vi "Demo of affinity propagation clustering algorithm.vi"() -> ()   [LabVIEW 2020]
doc: "An algorithm that exchanges messages about the similarity of pairs of data points speeds identification of representative examples in a complex data set, such as genes in DNA data."
uses:
  PLAIYDISPLAY/Display/Classification/2D/Predicted/Controls/PredictedParameter.ctl
  PLAIYDISPLAY/Display/_Controls/Style.ctl
  Model/Unsupervised/Cluster/AffinityPropagation/Controls/affinity_propagation_params.ctl
  Model/Unsupervised/Cluster/AffinityPropagation/AffinityPropagation.lvclass
  C:/Users/cipop/TDF Dropbox/2_Technologies de France/1 - Services et Etudes/PLAIY/2 - DEV/PLAIYLAB/code/Model/Model.lvclass
  Model/Unsupervised/Cluster/AffinityPropagation/AffinityPropagation.vi
  Preproc/Objet/3 - Model selection and evaluation/3.3 - Metrics and scoring/silhouette_score/Silhouette_Score.vi
  Preproc/Objet/3 - Model selection and evaluation/3.3 - Metrics and scoring/homogeneity_score/Homogeneity_Score.vi
  Preproc/Objet/3 - Model selection and evaluation/3.3 - Metrics and scoring/completeness_score/Completeness_Score.vi
  Preproc/Objet/3 - Model selection and evaluation/3.3 - Metrics and scoring/v_measure_score/V_Measure_Score.vi
  Preproc/Objet/3 - Model selection and evaluation/3.3 - Metrics and scoring/adjusted_rand_score/Adjusted_Rand_Score.vi
  Preproc/Objet/3 - Model selection and evaluation/3.3 - Metrics and scoring/adjusted_mutual_info_score/Adjusted_Mutual_Info_Score.vi
panel:
  in  "Local":T1
  out "Silhouette Coefficient":string
  out "Adjusted Mutual Information":string
  out "Adjusted Rand Index":string
  out "V-measure":string
  out "Completeness":string
  out "Homogeneity":string
  out "error out":errorcluster
  out "Plot":cluster{"X":dbl[], "Y":dbl[]}[](graph) caption="Estimated number of cluster: 3"
  out "labels":dbl[](array[numeric])
  out "n_clusters_":i32
  out "cluster_centers_indices":dbl[](array[numeric])
  in  "error in (no error) 2":errorcluster caption="entrée d'erreur (pas d'erreur)"
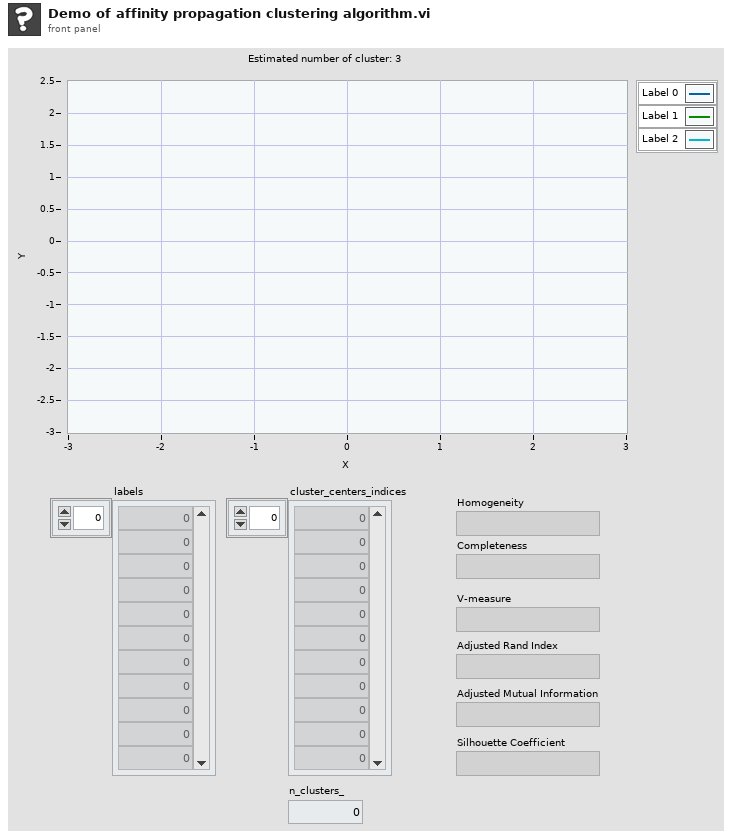
[diagram p1: front panel]
types:
  T1 = cluster{"X":dbl[][], "labels_true":dbl[], "labels_":dbl[]}
  T2 = cluster{"n_samples":i32[], "n_features":u32, "centers":i32[][], "cluster_std":dbl[], "centermin":dbl, "centermax":dbl, "shuffle":bool, "random_state":i32, "Returns":string}
  T3 = typedef "affinity_propagation_params.ctl" = cluster{"damping":dbl, "max_iter":i32, "convergence_iter":i32, "copy":bool, "preference":cluster{"preference_type":string, "preference_list":dbl[], "preference_float":dbl}, "affinity":string, "verbose":bool, "random_state":i32}
  T4 = typedef "Style.ctl" = enum16{"Empty circle", "Full circle", "Empty square", "Full square", "Cross"}
  T5 = typedef "PredictedParameter.ctl" = cluster{"Plot":refnum<vi>, "Data":cluster{"X":dbl[][], "Predict":dbl[][]}, "Indexe":cluster{"X":i32, "Y":i32}, "Point Property":cluster{"Style":T4, "Label Color":u32[]}}
  T6 = cluster{"metric":string, "sample_size":string, "random_state":i32}
  T7 = cluster{" 4DArray":cluster{"1":string[][], "2":string[][]}[], " 3DArray":cluster{"Tableau":string[][]}[], "Sparse Matrix 2DArray":string[][], " 2DArray":string[][], " 1DArray":string[]}
  T8 = typedef "affinity_propagation_attributes.ctl" = cluster{"cluster_centers_indices_":dbl[], "cluster_centers_":dbl[][], "labels_":dbl[], "affinity_matrix_":dbl[][], "n_iter_":dbl}
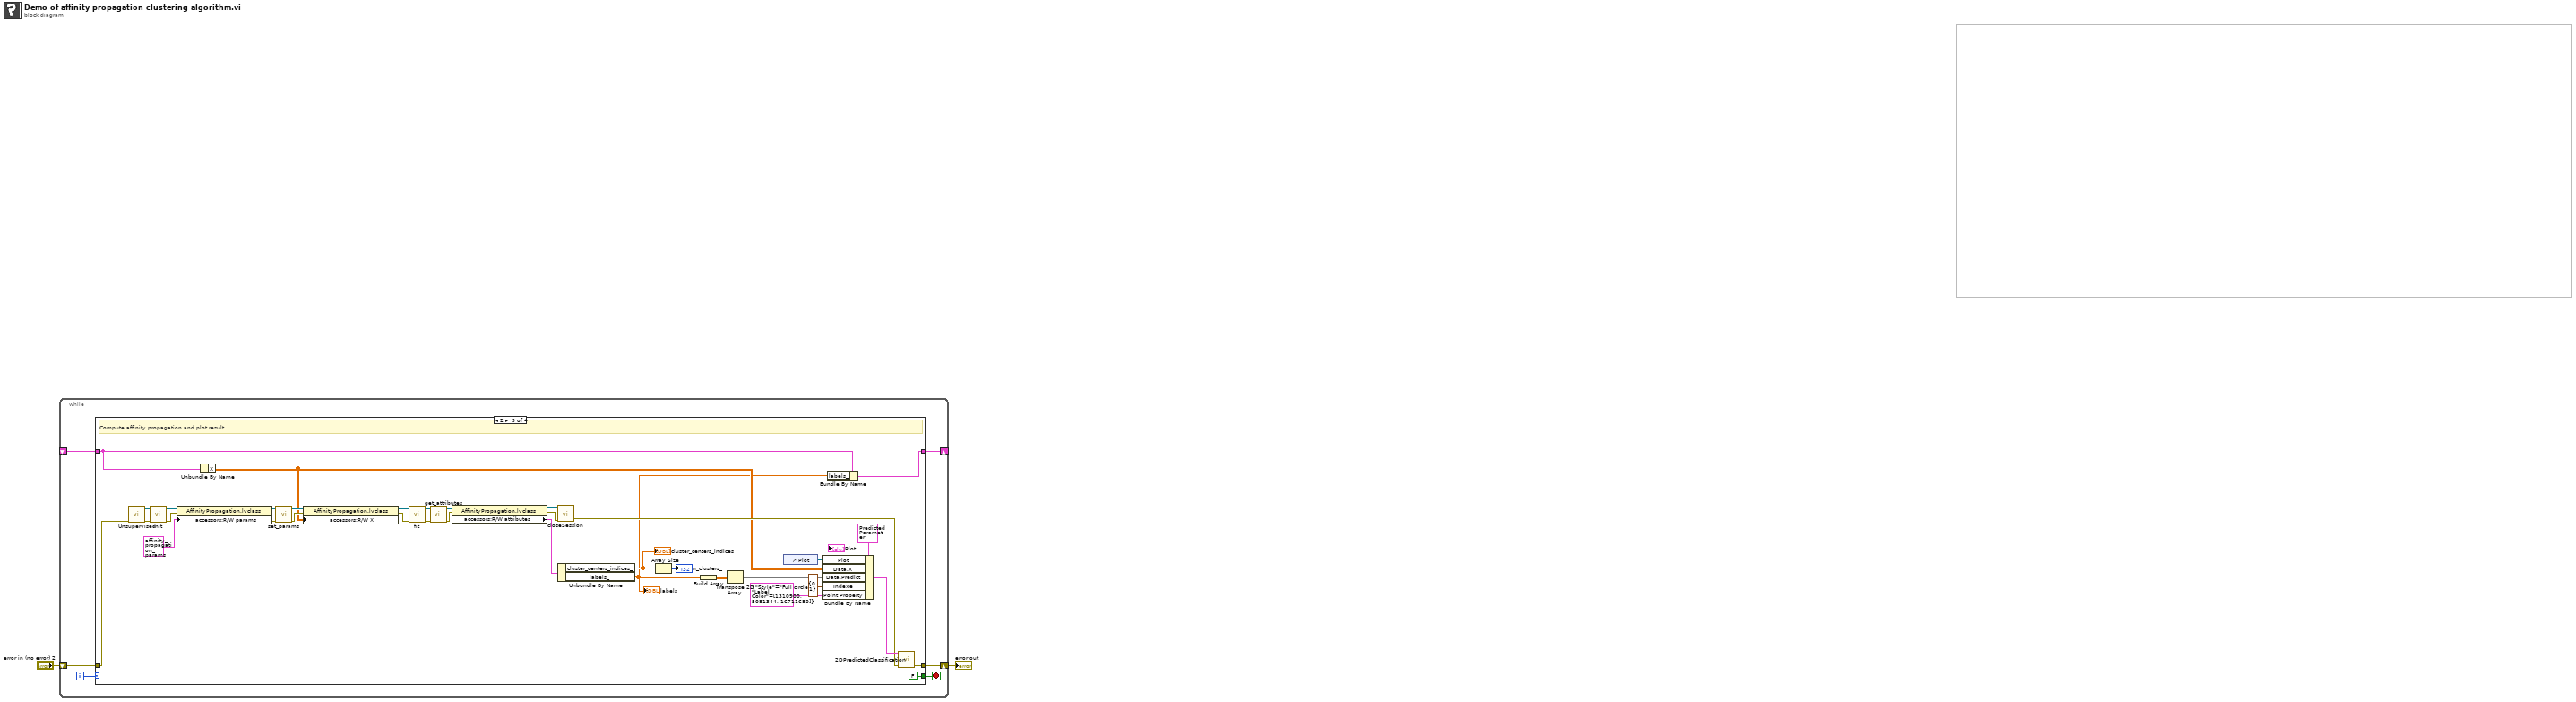
[diagram p0: block diagram]
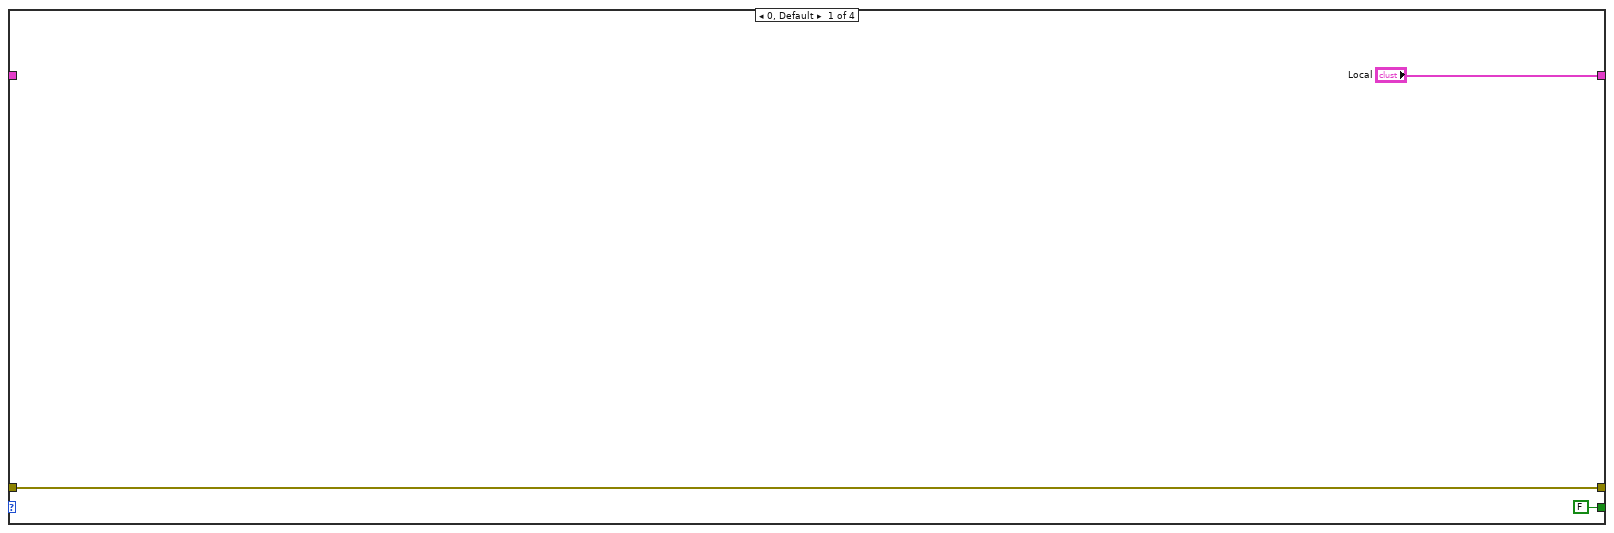
[diagram p2: hidden frame]
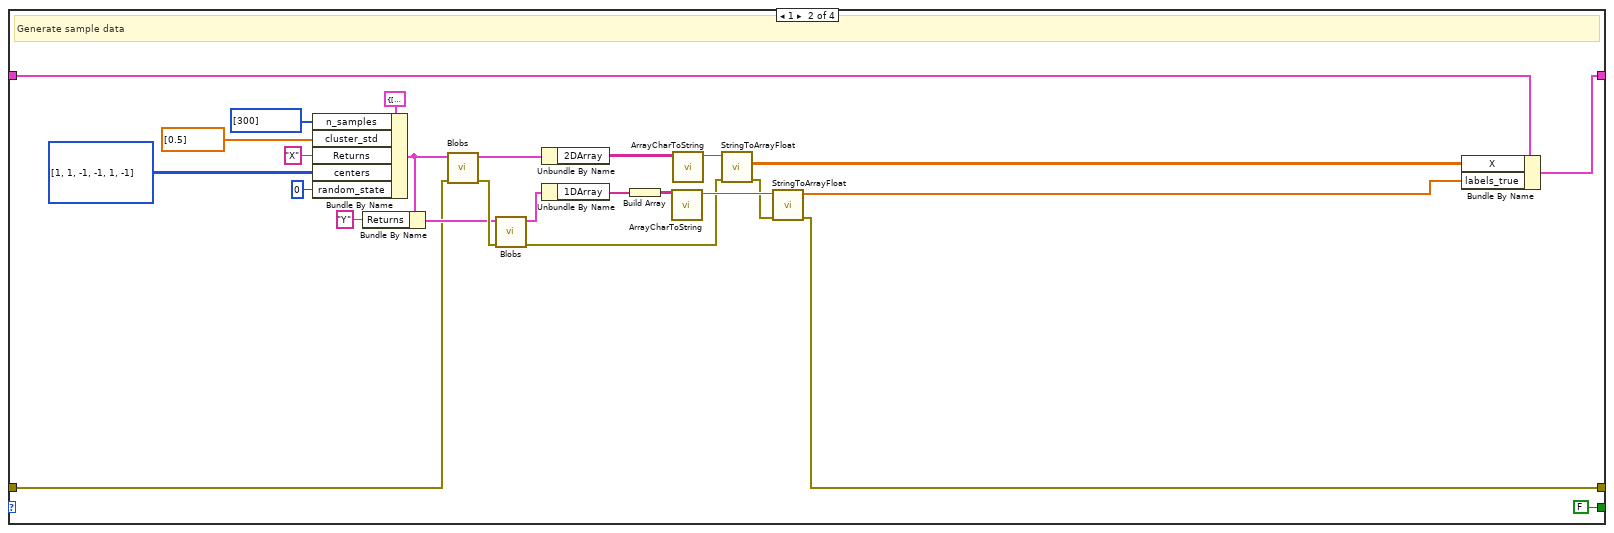
[diagram p3: hidden frame]
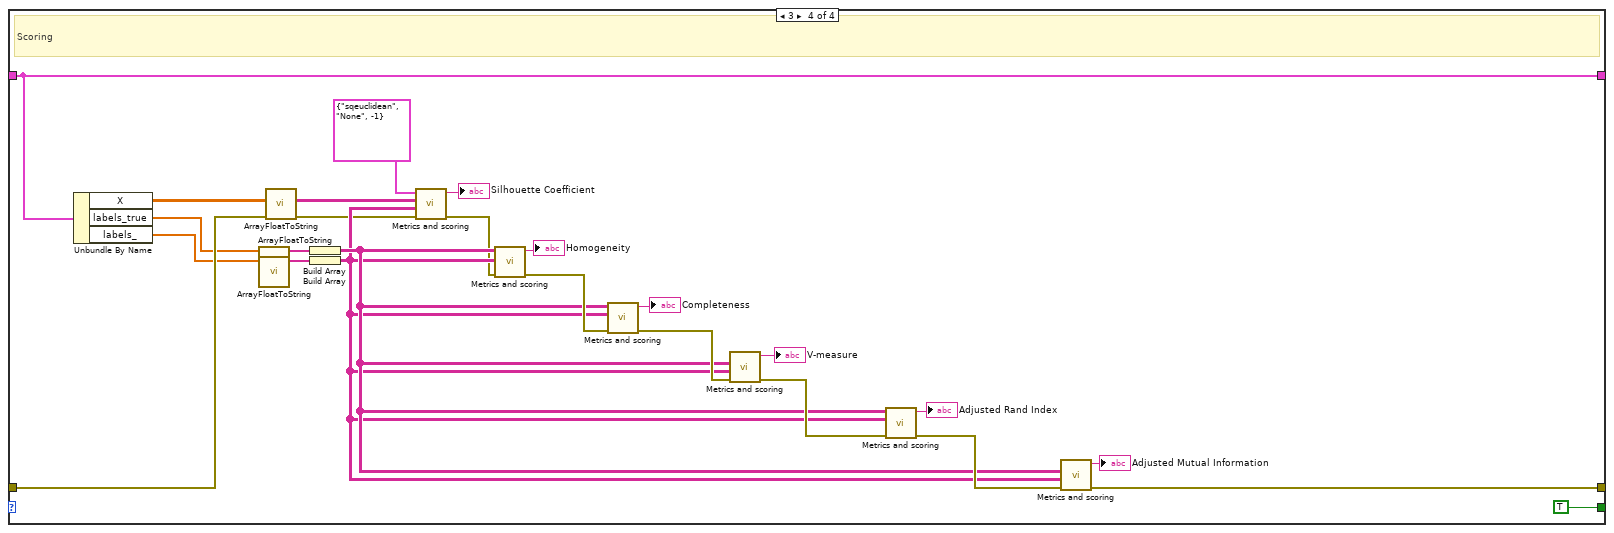
[diagram p4: hidden frame]
diagram:
  n1 = while {
    shift-right: [w6] -> w1
    shift-left: "error in (no error) 2" -> [w8]
    shift-right: [w4] -> _
    shift-left: _ -> [w3]
    i -> [w7]
    stop <- w5 stop-if-true
    n2 = case shown="2" w7 {
      tunnel: w8 -> [w10 w18 w60 w80]
      tunnel: [w10 w17 w43 w79] -> w6
      tunnel: [FALSE FALSE FALSE TRUE] -> w5
      tunnel: ["Local" w14 w38 w74] -> w4
      tunnel: w3 -> [_ w15 w40 w74]
      frame 0, Default {
      }
      frame 1 {
        # "Generate sample data"
        n3 = Bundle By Name(cluster=T2 {"n_samples"=[100], "n_features"=2, "centers"=[], "cluster_std"=[], "centermin"=-10.0, "centermax"=10.0, "shuffle"=TRUE, "random_state"=-1, "Returns"="X"} ("make_blobs"), "n_samples"=i32[] [300], "cluster_std"=dbl[] [0.5], "Returns"="X", "centers"=i32[][] [[1, 1], [-1, -1], [1, -1]], "random_state"=0) -> (w20:T2)
        n4 = Bundle By Name(cluster=w20, "Returns"="Y") -> (w31:T2)
        n5 = call "Blobs.vi"("error in (no error)"=w18, "make_blobs"=w20) -> ("error out"=w35:errorcluster, "Data"=w37:T7)  [unwired: 8 in]
        n6 = call "Blobs.vi"("error in (no error)"=w35, "make_blobs"=w31) -> ("error out"=w27:errorcluster, "Data"=w30:T7)  [unwired: 8 in]
        n7 = Unbundle By Name(w37) -> ("2DArray"=w23:string[][])
        n8 = Unbundle By Name(w30) -> ("1DArray"=w25:string[])
        n9 = Build Array(w25) -> (w24:string[][])
        n10 = call "ArrayCharToString.vi"("TAB"=w24) -> ("Instruction"=w28:string)  [unwired: 10 in]
        n11 = call "ArrayCharToString.vi"("TAB"=w23) -> ("Instruction"=w36:string)  [unwired: 10 in]
        n12 = call "StringToArrayFloat.vi"("entrée d'erreur (pas d'erreur)"=w27, "Return value"=w36) -> ("error IO"=w26:errorcluster, "2DArray"=w13:dbl[][])  [unwired: 7 in, 1 out]
        n13 = call "StringToArrayFloat.vi"("entrée d'erreur (pas d'erreur)"=w26, "Return value"=w28) -> ("error IO"=w17:errorcluster, "1DArray"=w12:dbl[])  [unwired: 7 in, 1 out]
        n14 = Bundle By Name(cluster=w15, "X"=w13, "labels_true"=w12) -> (w14:T1)
      }
      frame 2 {
        # "Compute affinity propagation and plot result"
        n15 = call-poly "Unsupervised.vi"("error in"=w60) -> ("error out"=w71:errorcluster, "out"=w72:refnum<class "AffinityPropagation.lvclass">)  [unwired: 9 in]
        n16 = call-dynamic "init.vi"("error in (no error)"=w71, "Model en entrée"=w72) -> ("error out"=w63:errorcluster, "Model en sortie"=w67:refnum<class "AffinityPropagation.lvclass">)  [unwired: 8 in]
        n17 = property class="AffinityPropagation.lvclass"(reference=w67, error in=w63, "accessors:R/W params"=T3 {"damping"=0.5, "max_iter"=200, "convergence_iter"=15, "copy"=TRUE, "preference"={"preference_type"="float", "preference_list"=[], "preference_float"=-50.0}, "affinity"="euclidean", "verbose"=FALSE, "random_state"=0} ("R/W params")) -> (reference out=w66:refnum<class "AffinityPropagation.lvclass">, error out=w68:errorcluster)
        n18 = Unbundle By Name(w40) -> ("X"=w41:dbl[][])
        n19 = call-dynamic "set_params.vi"("error in (no error)"=w68, "AffinityPropagation.lvclass 2"=w66) -> ("error out"=w64:errorcluster, "AffinityPropagation.lvclass"=w65:refnum<class "AffinityPropagation.lvclass">)  [unwired: 8 in]
        n20 = property class="AffinityPropagation.lvclass"(reference=w65, error in=w64, "accessors:R/W X"=w41) -> (reference out=w70:refnum<class "AffinityPropagation.lvclass">, error out=w69:errorcluster)
        n21 = call-dynamic "fit.vi"("error in (no error)"=w69, "AffinityPropagation.lvclass 2"=w70) -> ("error out"=w61:errorcluster, "AffinityPropagation.lvclass"=w62:refnum<class "AffinityPropagation.lvclass">)  [unwired: 8 in]
        n22 = call-dynamic "get_attributes.vi"("error in (no error)"=w61, "AffinityPropagation.lvclass 2"=w62) -> ("error out"=w45:errorcluster, "AffinityPropagation.lvclass"=w46:refnum<class "AffinityPropagation.lvclass">)  [unwired: 8 in]
        n23 = property class="AffinityPropagation.lvclass"(reference=w46, error in=w45) -> (reference out=w58:refnum<class "AffinityPropagation.lvclass">, error out=w57:errorcluster, "accessors:R/W attributes"=w56:T8)
        n24 = call-dynamic "closeSession.vi"("error in"=w57, "Python en entrée"=w58) -> ("error out"=w44:errorcluster)  [unwired: 8 in, 1 out]
        n25 = Unbundle By Name(w56) -> ("cluster_centers_indices_"=w55:dbl[], "labels_"=w39:dbl[])
        "cluster_centers_indices" <- w55
        "labels" <- w39
        n26 = Array Size(array=w55) -> (size(s)=→"n_clusters_":i32)
        n27 = Build Array(w39) -> (w49:dbl[][])
        n28 = Transpose 2D Array(2D array=w49) -> (transposed array=w48:dbl[][])
        n29 = control-ref of="Plot"() -> (w52:refnum<vi>)
        n30 = Bundle By Name(cluster=T5 {"Plot"=refnum, "Data"={"X"=[], "Predict"=[]}, "Indexe"={"X"=0, "Y"=1}, "Point Property"={"Style"=enum."Full circle", "Label Color"=[8978528, 4367871, 1985280]}} ("Parameters"), "Plot"=w52, "Data.X"=w41, "Data.Predict"=w48, "Indexe"=cluster{"X":i32, "Y":i32} {"X"=0, "Y"=1}, "Point Property"=cluster{"Style":T4, "Label Color":u32[]} {"Style"=enum."Full circle", "Label Color"=[1310900, 5081344, 16711680]}) -> (w51:T5)
        n31 = Bundle By Name(cluster=w40, "labels_"=w39) -> (w38:T1)
        n32 = call "2DPredictedClassification.vi"("error in"=w44, "Parameters"=w51) -> ("error out"=w43:errorcluster)  [unwired: 9 in]
      }
      frame 3 {
        # "Scoring"
        n33 = Unbundle By Name(w74) -> ("X"=w77:dbl[][], "labels_true"=w76:dbl[], "labels_"=w75:dbl[])
        n34 = call "ArrayFloatToString.vi"("1D Data"=w76) -> ("Array"=w84:string[])  [unwired: 9 in, 1 out]
        n35 = call "ArrayFloatToString.vi"("1D Data"=w75) -> ("Array"=w95:string[])  [unwired: 9 in, 1 out]
        n36 = call "ArrayFloatToString.vi"("2D Data"=w77) -> ("Array"=w73:string[][])  [unwired: 9 in, 1 out]
        n37 = Build Array(w84) -> (w83:string[][])
        n38 = Build Array(w95) -> (w82:string[][])
        n39 = call-poly "Metrics and scoring.vi"("error in (no error)"=w80, "labels"=w82, "X"=w73, "silhouette_score"=T6 {"metric"="sqeuclidean", "sample_size"="None", "random_state"=-1}) -> ("error out"=w81:errorcluster, "Score"=→"Silhouette Coefficient":string)  [unwired: 6 in]
        n40 = call-poly "Metrics and scoring.vi"("error in (no error)"=w81, "labels_pred"=w82, "labels_true"=w83) -> ("error out"=w96:errorcluster, "Score"=→"Homogeneity":string)  [unwired: 7 in]
        n41 = call-poly "Metrics and scoring.vi"("error in (no error)"=w96, "labels_pred"=w82, "labels_true"=w83) -> ("error out"=w92:errorcluster, "Score"=→"Completeness":string)  [unwired: 7 in]
        n42 = call-poly "Metrics and scoring.vi"("error in (no error)"=w92, "labels_pred"=w82, "labels_true"=w83) -> ("error out"=w90:errorcluster, "Score"=→"V-measure":string)  [unwired: 7 in]
        n43 = call-poly "Metrics and scoring.vi"("error in"=w90, "labels_pred"=w82, "labels_true"=w83) -> ("error out"=w88:errorcluster, "Score"=→"Adjusted Rand Index":string)  [unwired: 7 in]
        n44 = call-poly "Metrics and scoring.vi"("error in"=w88, "labels_pred"=w82, "labels_true"=w83) -> ("error out"=w79:errorcluster, "Score"=→"Adjusted Mutual Information":string)  [unwired: 7 in]
      }
    }
  }
  "error out" <- w1
